vi "Analyze.vi"(9 "Threshold (rms)":dbl, 10 "Data (1D DBL)":dbl[](array[numeric])) -> (1 "Threshold Exceeded?":bool, 2 "RMS Result":dbl)   [LabVIEW 2020]
uses:
  <vilib>/Analysis/5stat.llb/RMS (DBL).vi
  <vilib>/Analysis/NI_AALPro.lvlib
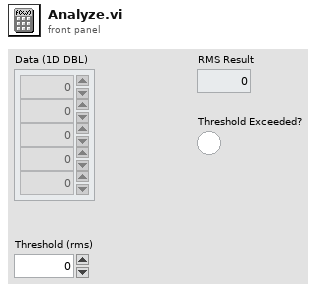
[diagram p1: front panel]
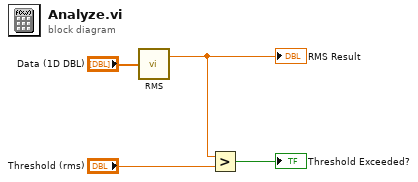
[diagram p0: block diagram]
diagram:
  n1 = call-poly <vilib>:"RMS.vi"("X"="Data (1D DBL)") -> ("rms value"=w2:dbl)  [unwired: 1 out]
  "RMS Result" <- w2
  n2 = Greater?(x=w2, y="Threshold (rms)") -> (0:→"Threshold Exceeded?":bool)
